vi "solar_voy_def Export (Mods_Convert).vi"(10 "CMD":enum8{"CMD", "TLM"}(ring), 11 "CONVERSION":T1) -> (3 "CONVERSION_DEF":string)   [LabVIEW 2018]
doc: "This exports a COSMOS conversion modifier to string."
uses:
  solar_voy_def_ctl MODIFIERS CONVERSION.ctl
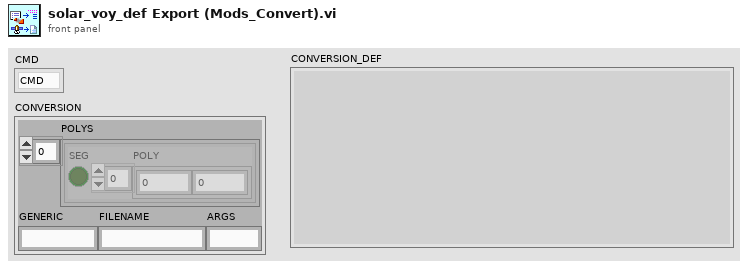
[diagram p1: front panel]
types:
  T1 = typedef "solar_voy_def_ctl MODIFIERS CONVERSION.ctl" = cluster{"GENERIC":string, "FILENAME":string, "ARGS":string, "POLYS":cluster{"SEG":bool, "POLY":dbl[]}[]}
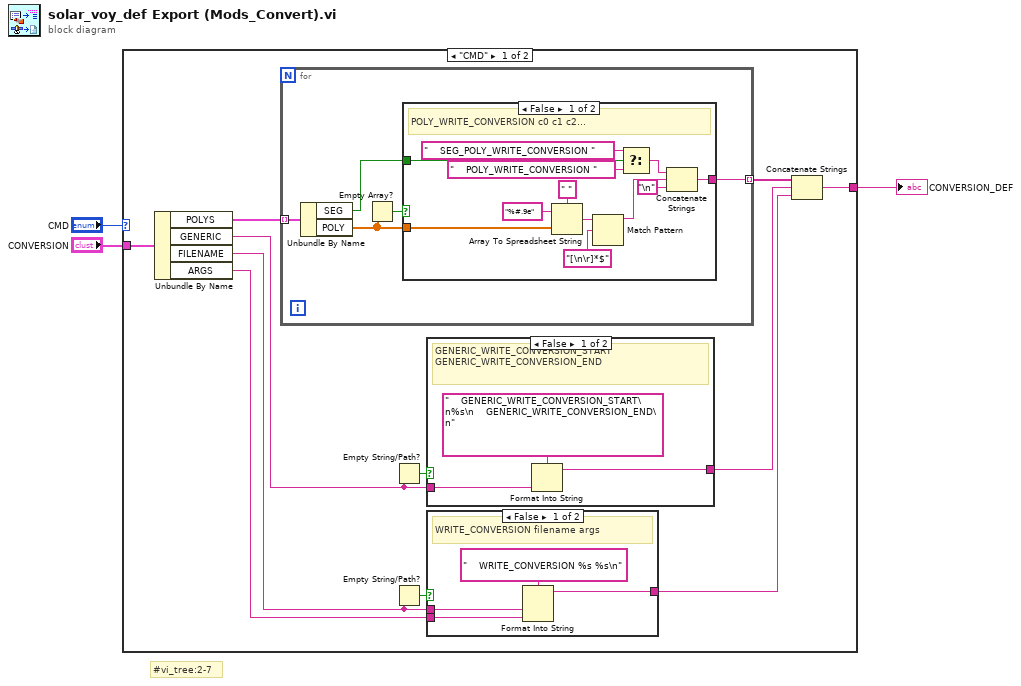
[diagram p0: block diagram]
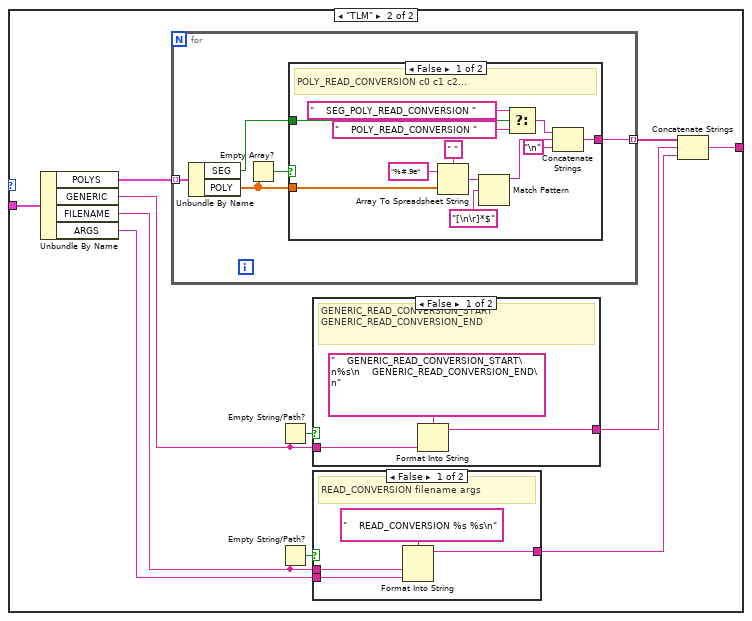
[diagram p5: hidden frame]
diagram:
  # "#vi_tree:2-7"
  n1 = case shown="\"CMD\"" "CMD" {
    tunnel: [w14 w49] -> w3
    tunnel: "CONVERSION" -> [w5 w40]
    frame "CMD" {
      n2 = Unbundle By Name(w5) -> ("POLYS"=w4:cluster{"SEG":bool, "POLY":dbl[]}[], "GENERIC"=w6:string, "FILENAME"=w9:string, "ARGS"=w10:string)
      n3 = for {
        tunnel: [w19] -> w11 mode=indexing
        tunnel: w4 -> [w17] mode=indexing
        n4 = Unbundle By Name(w17) -> ("SEG"=w16:bool, "POLY"=w15:dbl[])
        n5 = Empty Array?(array=w15) -> (empty?=w18:bool)
        n6 = case shown="False" w18 {
          tunnel: w15 -> [w31 _]
          tunnel: [w24 _] -> w19
          tunnel: w16 -> [w23 _]
          frame False {
            # "POLY_WRITE_CONVERSION c0 c1 c2..."
            n7 = Array To Spreadsheet String(delimiter (Tab)=" ", array=w31, 3:"%#.9e" ("format string")) -> (spreadsheet string=w27:string)
            n8 = Match Pattern(string=w27, regular expression="[\n\r]*$") -> (before substring=w26:string)  [unwired: 1 in, 3 out]
            n9 = Select(t="    SEG_POLY_WRITE_CONVERSION ", s=w23, f="    POLY_WRITE_CONVERSION ") -> (s? t:f=w20:string)
            n10 = Concatenate Strings(w20, w26, "\n" ("Line Feed Constant")) -> (w24:string)
          }
          frame True {
          }
        }
      }
      n11 = Empty String/Path?(string/path=w6) -> (empty?=w7:bool)
      n12 = Empty String/Path?(string/path=w9) -> (empty?=w8:bool)
      n13 = case shown="False" w7 {
        tunnel: w6 -> [w37 _]
        tunnel: [w36 _] -> w12
        frame False {
          # "GENERIC_WRITE_CONVERSION_START\nGENERIC_WRITE_CONVERSION_END"
          n14 = Format Into String(format string="    GENERIC_WRITE_CONVERSION_START\n%s\n    GENERIC_WRITE_CONVERSION_END\n", w37) -> (resulting string=w36:string)  [unwired: 2 in, 1 out]
        }
        frame True {
        }
      }
      n15 = case shown="False" w8 {
        tunnel: w9 -> [w34 _]
        tunnel: [w33 _] -> w13
        tunnel: w10 -> [w32 _]
        frame False {
          # "WRITE_CONVERSION filename args"
          n16 = Format Into String(format string="    WRITE_CONVERSION %s %s\n", w34, w32) -> (resulting string=w33:string)  [unwired: 2 in, 1 out]
        }
        frame True {
        }
      }
      n17 = Concatenate Strings(w11, w12, w13) -> (w14:string)
    }
    frame "TLM" {
      n18 = Unbundle By Name(w40) -> ("POLYS"=w39:cluster{"SEG":bool, "POLY":dbl[]}[], "GENERIC"=w41:string, "FILENAME"=w44:string, "ARGS"=w45:string)
      n19 = for {
        tunnel: [w54] -> w46 mode=indexing
        tunnel: w39 -> [w52] mode=indexing
        n20 = Unbundle By Name(w52) -> ("SEG"=w51:bool, "POLY"=w50:dbl[])
        n21 = Empty Array?(array=w50) -> (empty?=w53:bool)
        n22 = case shown="False" w53 {
          tunnel: w50 -> [w66 _]
          tunnel: [w59 _] -> w54
          tunnel: w51 -> [w58 _]
          frame False {
            # "POLY_READ_CONVERSION c0 c1 c2..."
            n23 = Array To Spreadsheet String(delimiter (Tab)=" ", array=w66, 3:"%#.9e" ("format string")) -> (spreadsheet string=w62:string)
            n24 = Match Pattern(string=w62, regular expression="[\n\r]*$") -> (before substring=w61:string)  [unwired: 1 in, 3 out]
            n25 = Select(t="    SEG_POLY_READ_CONVERSION ", s=w58, f="    POLY_READ_CONVERSION ") -> (s? t:f=w55:string)
            n26 = Concatenate Strings(w55, w61, "\n" ("Line Feed Constant")) -> (w59:string)
          }
          frame True {
          }
        }
      }
      n27 = Empty String/Path?(string/path=w41) -> (empty?=w42:bool)
      n28 = Empty String/Path?(string/path=w44) -> (empty?=w43:bool)
      n29 = case shown="False" w42 {
        tunnel: w41 -> [w72 _]
        tunnel: [w71 _] -> w47
        frame False {
          # "GENERIC_READ_CONVERSION_START\nGENERIC_READ_CONVERSION_END"
          n30 = Format Into String(format string="    GENERIC_READ_CONVERSION_START\n%s\n    GENERIC_READ_CONVERSION_END\n", w72) -> (resulting string=w71:string)  [unwired: 2 in, 1 out]
        }
        frame True {
        }
      }
      n31 = case shown="False" w43 {
        tunnel: w44 -> [w69 _]
        tunnel: [w68 _] -> w48
        tunnel: w45 -> [w67 _]
        frame False {
          # "READ_CONVERSION filename args"
          n32 = Format Into String(format string="    READ_CONVERSION %s %s\n", w69, w67) -> (resulting string=w68:string)  [unwired: 2 in, 1 out]
        }
        frame True {
        }
      }
      n33 = Concatenate Strings(w46, w47, w48) -> (w49:string)
    }
  }
  "CONVERSION_DEF" <- w3
